vi "SLSC Add or Remove Channels.vi"(0 "Section Ref in":T1 format="%.0x", 1 "Properties":string="Properties", 2 "Command Channel":string="Commands", 3 "Physical Channels":string="Physical Channels", 5 "Property tree":string[](array[string]), 7 "Add or Remove":bool, 9 "SLSC EDS module in":T2, 11 "error in (no error)":errorcluster, 12 "Enums":T3[](array[typedef])) -> (4 "Section Ref out":T1 format="%.0x", 15 "error out":errorcluster)   [LabVIEW 2019, in "SLSC EDS System Explorer.lvlib"]
uses:
  SLSC EDS System Explorer.lvlib
  SLSC EDS API/JSON parsing/enum.ctl
  <vilib>/NI VeriStand/Custom Device API/Custom Device Item Ref.ctl
  SLSC EDS API/JSON parsing/EDSjsonStructure.ctl
  SLSC EDS API/JSON parsing/property.ctl
  SLSC EDS API/JSON parsing/command.ctl
  SLSC EDS API/JSON parsing/scale.ctl
  SLSC EDS API/JSON parsing/physicalChannel.ctl
  SLSC EDS API/JSON parsing/register.ctl
  <vilib>/NI VeriStand/Custom Device Tools/Custom Device Utility Library/NI VeriStand - Search for Item by Name.vi
  <vilib>/NI VeriStand/Custom Device Tools/Custom Device Utility Library/NI VeriStand - Search for All Items by Name.vi
  <vilib>/NI VeriStand/Custom Device Tools/Custom Device Utility Library/Custom Device Utility Library.lvlib
  <vilib>/NI VeriStand/Custom Device API/Custom Device API.lvlib
  SLSC UI API/SLSC Tree Control.lvlib
panel:
  # "not working\nregisterMap->registers->initialValue"
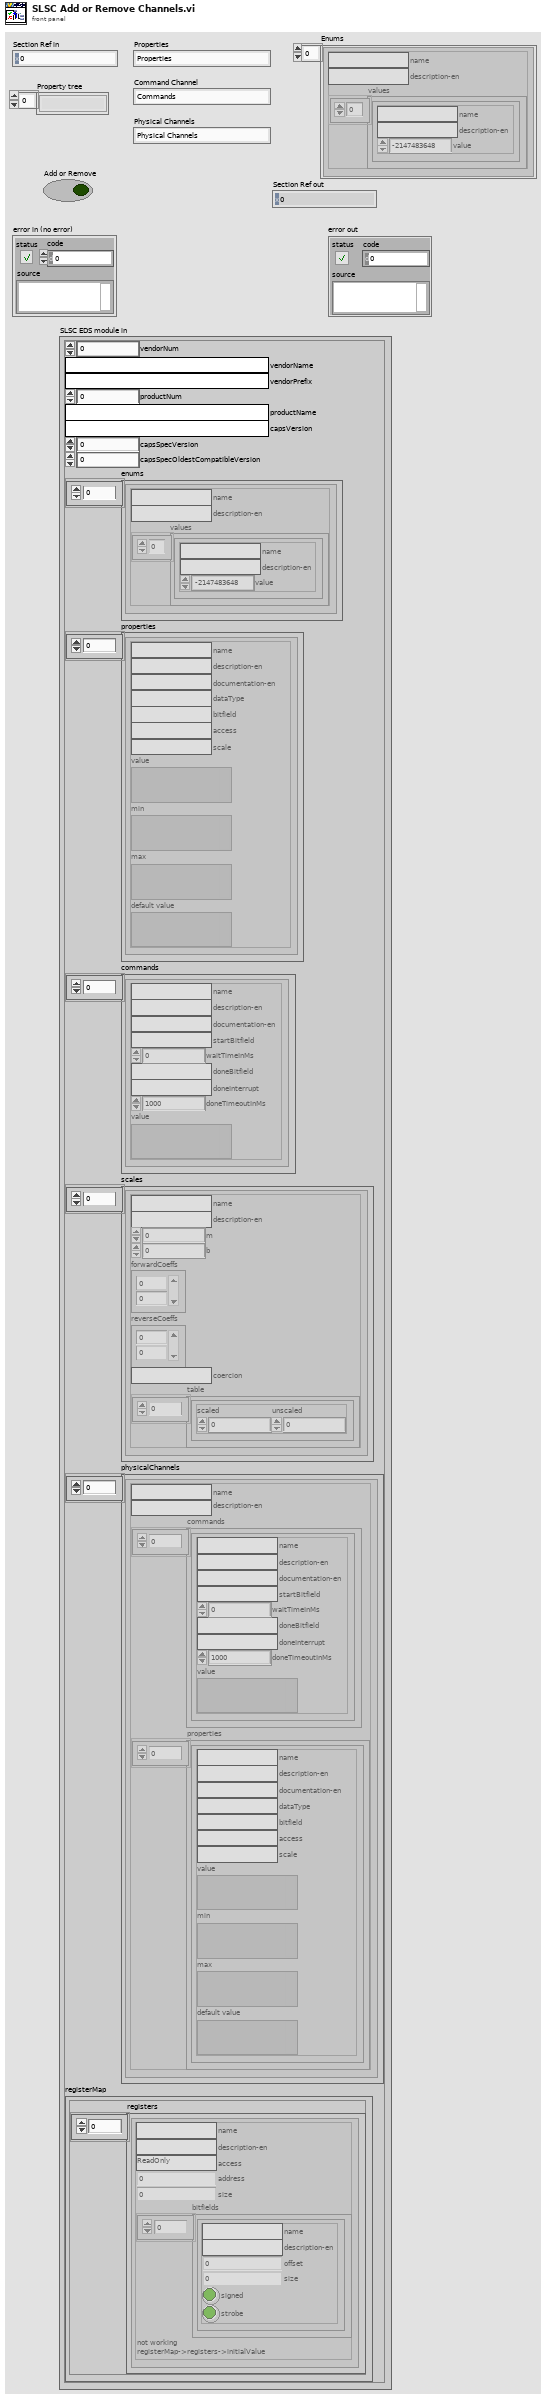
[diagram p1: front panel]
types:
  T1 = typedef "Custom Device API.lvlib/Custom Device Item Ref.ctl" = u64
  T2 = typedef "EDSjsonStructure.ctl" = cluster{"vendorNum":u32, "vendorName":string, "vendorPrefix":string, "productNum":u32, "productName":string, "capsVersion":string, "capsSpecVersion":u32, "capsSpecOldestCompatibleVersion":u32, "enums":T3[], "properties":T4[], "commands":T5[], "scales":T6[], "physicalChannels":T7[], "registerMap":cluster{"registers":T8[]}}
  T3 = typedef "enum.ctl" = cluster{"name":string, "description-en":string, "values":cluster{"name":string, "description-en":string, "value":i32}[]}
  T4 = typedef "property.ctl" = cluster{"name":string, "description-en":string, "documentation-en":string, "dataType":string, "bitfield":string, "access":string, "scale":string, "value":variant, "min":variant, "max":variant, "default value":variant}
  T5 = typedef "command.ctl" = cluster{"name":string, "description-en":string, "documentation-en":string, "startBitfield":string, "waitTimeInMs":i32, "doneBitfield":string, "doneInterrupt":string, "doneTimeoutInMs":i32, "value":variant}
  T6 = typedef "scale.ctl" = cluster{"name":string, "description-en":string, "m":dbl, "b":dbl, "forwardCoeffs":dbl[], "reverseCoeffs":dbl[], "coercion":string, "table":cluster{"scaled":dbl, "unscaled":dbl}[]}
  T7 = typedef "physicalChannel.ctl" = cluster{"name":string, "description-en":string, "commands":T5[], "properties":T4[]}
  T8 = typedef "register.ctl" = cluster{"name":string, "description-en":string, "access":string, "address":u32, "size":u32, "bitfields":cluster{"name":string, "description-en":string, "offset":u32, "size":u32, "signed":bool, "strobe":bool}[]}
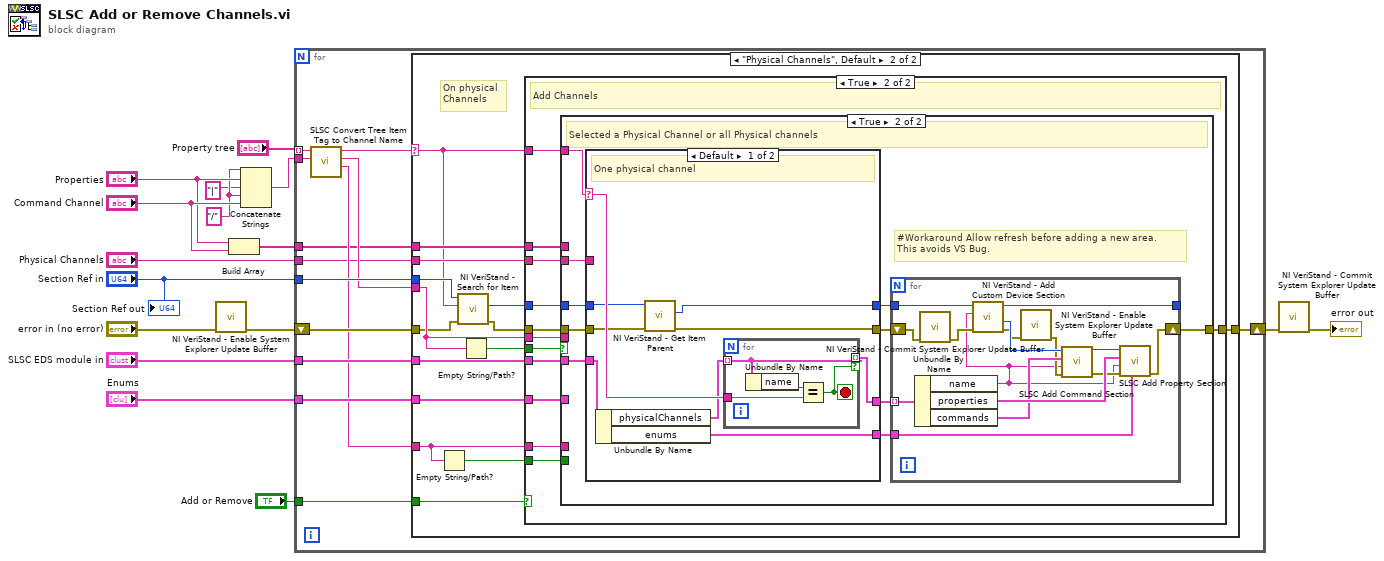
[diagram p0: block diagram]
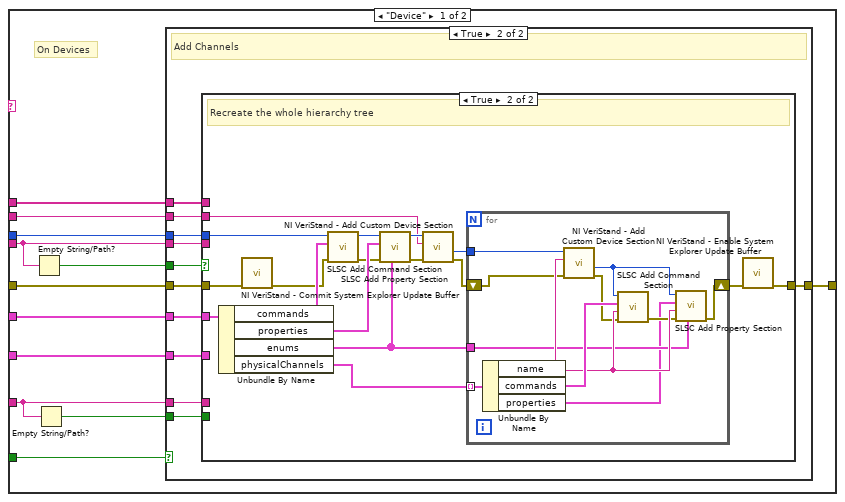
[diagram p2: hidden frame]
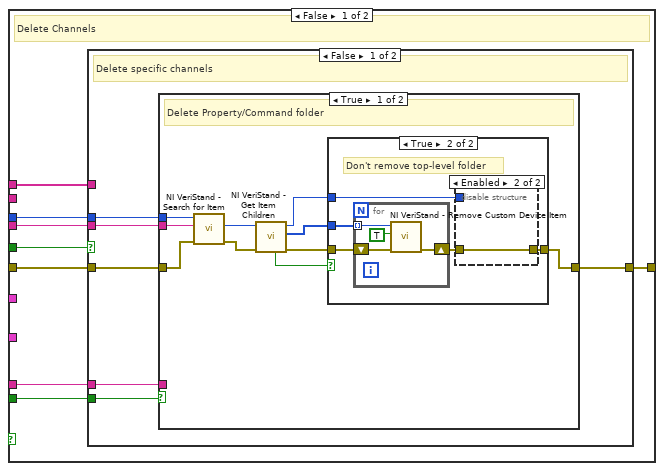
[diagram p3: hidden frame]
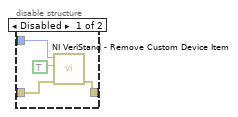
[diagram p5: hidden frame]
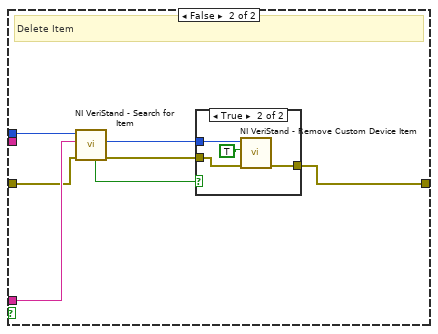
[diagram p6: hidden frame]
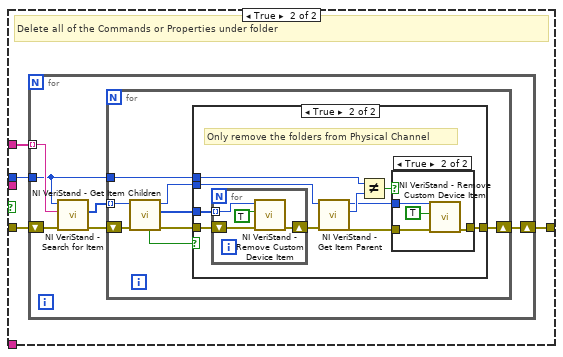
[diagram p8: hidden frame]
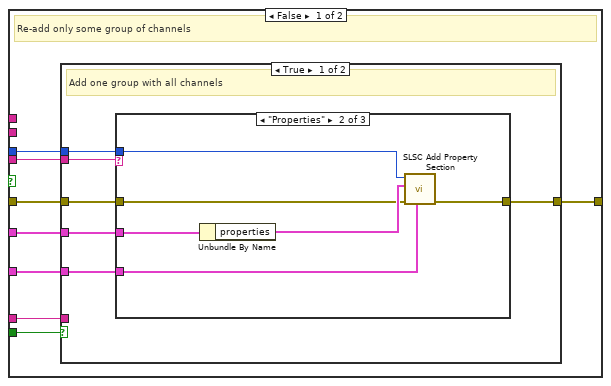
[diagram p11: hidden frame]
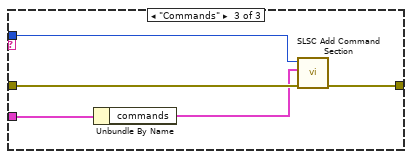
[diagram p13: hidden frame]
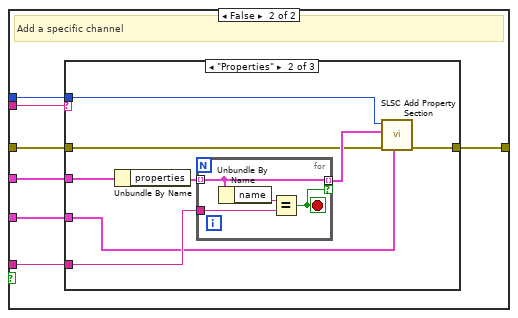
[diagram p14: hidden frame]
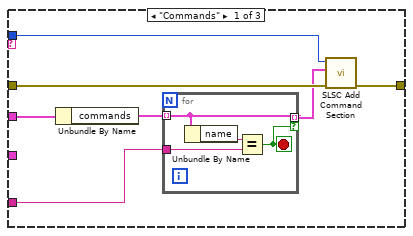
[diagram p15: hidden frame]
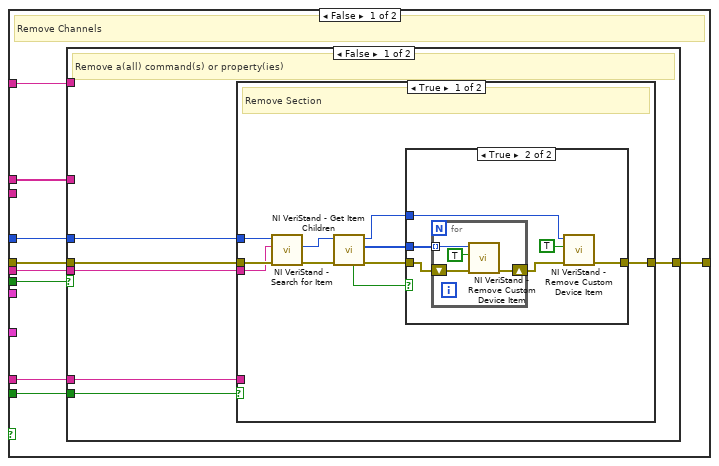
[diagram p17: hidden frame]
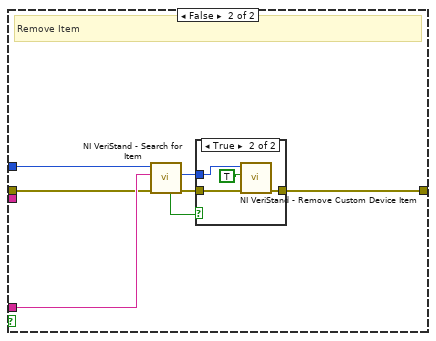
[diagram p19: hidden frame]
diagram:
  w6 = "/" ("string")
  n1 = call <vilib>:"NI VeriStand - Enable System Explorer Update Buffer.vi"("error in (no error)"="error in (no error)") -> ("error out"=w10:errorcluster)  [unwired: 10 in]
  n2 = Build Array("Properties", "Command Channel") -> (w8:string[])
  n3 = Concatenate Strings(w6, "Properties", "|" ("string"), w6, "Command Channel") -> (w4:string)
  n4 = for {
    tunnel: "Property tree" -> [w21] mode=indexing
    tunnel: w4 -> [w28]
    tunnel: "Section Ref in" -> [w27]
    shift-right: [w25] -> w15
    shift-left: w10 -> [w26]
    tunnel: "Add or Remove" -> [w24]
    tunnel: "SLSC EDS module in" -> [w23]
    tunnel: "Enums" -> [w22]
    tunnel: w8 -> [w18]
    tunnel: "Physical Channels" -> [w17]
    n5 = call "SLSC Convert Tree Item Tag to Channel Name.vi"("Type of Item"=w28, "Item String"=w21) -> ("Item Name"=w20:string, "Type of Item"=w19:string, "Device/Physical Channel"=w29:string)  [unwired: 7 in]
    n6 = case shown="\"Physical Channels\", Default" w29 {
      selector: w29 -> [_ w227]
      tunnel: w20 -> [w35 w237]
      tunnel: w27 -> [w41 w231]
      tunnel: w26 -> [w40 w229]
      tunnel: [w39 w241] -> w25
      tunnel: w24 -> [w38 w240]
      tunnel: w23 -> [w37 w239]
      tunnel: w22 -> [w36 w238]
      tunnel: w19 -> [w33 w235]
      tunnel: w18 -> [w31 w233]
      tunnel: w17 -> [w30 w232]
      frame "Device" {
        # "On Devices"
        n7 = Empty String/Path?(string/path=w33) -> (empty?=w32:bool)
        n8 = Empty String/Path?(string/path=w35) -> (empty?=w34:bool)
        n9 = case shown="True" w38 {
          tunnel: w41 -> [w49 w141]
          tunnel: w35 -> [w48 w138]
          tunnel: w40 -> [w47 w140]
          tunnel: [w46 w137] -> w39
          tunnel: w37 -> [_ w139]
          tunnel: w36 -> [_ w136]
          tunnel: w33 -> [w44 w134]
          tunnel: w34 -> [w45 w135]
          tunnel: w32 -> [w43 w133]
          tunnel: w31 -> [w42 w131]
          tunnel: w30 -> [_ w132]
          frame False {
            # "Delete Channels"
            n10 = case shown="False" w43 {
              tunnel: w49 -> [w55 w96]
              tunnel: w48 -> [w54 _]
              tunnel: w47 -> [w50 w94]
              tunnel: [w51 w93] -> w46
              tunnel: w45 -> [w53 _]
              tunnel: w44 -> [w52 _]
              tunnel: w42 -> [_ w95]
              frame False {
                # "Delete specific channels"
                n11 = case shown="True" w53 {
                  tunnel: w55 -> [w65 w87]
                  tunnel: w54 -> [_ w86]
                  tunnel: w50 -> [w64 w84]
                  tunnel: [w63 w82] -> w51
                  tunnel: w52 -> [w57 _]
                  frame True {
                    # "Delete Property/Command folder"
                    n12 = call-poly <vilib>:"NI VeriStand - Search for Item.vi"("error in"=w64, "Item Name"=w57, "Section Ref in"=w65) -> ("error out"=w59:errorcluster, "Item Ref"=w62:T1)  [unwired: 5 in, 2 out]
                    n13 = call <vilib>:"NI VeriStand - Get Item Children.vi"("error in (no error)"=w59, "Item Ref in"=w62) -> ("error out"=w58:errorcluster, "Child Refs"=w61:T1[], "Item Ref out"=w56:T1, "Found"=w60:bool)  [unwired: 6 in]
                    n14 = case shown="True" w60 {
                      tunnel: w61 -> [_ w71]
                      tunnel: w58 -> [w66 w70]
                      tunnel: [w66 w68] -> w63
                      tunnel: w56 -> [_ w67]
                      frame False {
                      }
                      frame True {
                        # "Don't remove top-level folder"
                        n15 = for {
                          tunnel: w71 -> [w80] mode=indexing
                          shift-right: [w78] -> w69
                          shift-left: w70 -> [w79]
                          n16 = call <vilib>:"NI VeriStand - Remove Custom Device Item.vi"("error in (no error)"=w79, "Force Delete (F)"=TRUE, "Item Ref in"=w80) -> ("error out"=w78:errorcluster)  [unwired: 7 in, 1 out]
                        }
                        n17 = disable-structure shown="Enabled" {
                          disable-tunnel: w69 -> [w74 w76]
                          disable-tunnel: [w73 w76] -> w68
                          disable-tunnel: w67 -> [w72 _]
                          frame Disabled {
                            n18 = call <vilib>:"NI VeriStand - Remove Custom Device Item.vi"("error in (no error)"=w74, "Force Delete (F)"=TRUE, "Item Ref in"=w72) -> ("error out"=w73:errorcluster)  [unwired: 7 in, 1 out]
                          }
                          frame Enabled {
                          }
                        }
                      }
                    }
                  }
                  frame False {
                    # "Delete Item"
                    n19 = call-poly <vilib>:"NI VeriStand - Search for Item.vi"("error in"=w84, "Item Name"=w86, "Section Ref in"=w87) -> ("error out"=w83:errorcluster, "Item Ref"=w85:T1, "Found"=w81:bool)  [unwired: 5 in, 1 out]
                    n20 = case shown="True" w81 {
                      tunnel: w85 -> [_ w92]
                      tunnel: w83 -> [w88 w91]
                      tunnel: [w88 w90] -> w82
                      frame False {
                      }
                      frame True {
                        n21 = call <vilib>:"NI VeriStand - Remove Custom Device Item.vi"("error in (no error)"=w91, "Force Delete (F)"=TRUE, "Item Ref in"=w92) -> ("error out"=w90:errorcluster)  [unwired: 7 in, 1 out]
                      }
                    }
                  }
                }
              }
              frame True {
                # "Delete all of the Commands or Properties under folder"
                n22 = for {
                  tunnel: w96 -> [w97]
                  tunnel: w95 -> [w99] mode=indexing
                  shift-right: [w98] -> w93
                  shift-left: w94 -> [w102]
                  n23 = call-poly <vilib>:"NI VeriStand - Search for Item.vi"("error in"=w102, "Item Name"=w99, "Section Ref in"=w97) -> ("error out"=w100:errorcluster, "Item Refs"=w101:T1[])  [unwired: 5 in, 2 out]
                  n24 = for {
                    tunnel: w101 -> [w110] mode=indexing
                    shift-right: [w105] -> w98
                    shift-left: w100 -> [w107]
                    tunnel: w97 -> [w103]
                    n25 = call <vilib>:"NI VeriStand - Get Item Children.vi"("error in (no error)"=w107, "Item Ref in"=w110) -> ("error out"=w106:errorcluster, "Child Refs"=w109:T1[], "Item Ref out"=w104:T1, "Found"=w108:bool)  [unwired: 6 in]
                    n26 = case shown="True" w108 {
                      tunnel: w109 -> [_ w121]
                      tunnel: w106 -> [w111 w120]
                      tunnel: [w111 w119] -> w105
                      tunnel: w104 -> [_ w118]
                      tunnel: w103 -> [_ w114]
                      frame False {
                      }
                      frame True {
                        # "Only remove the folders from Physical Channel"
                        n27 = for {
                          tunnel: w121 -> [w127] mode=indexing
                          shift-right: [w129] -> w117
                          shift-left: w120 -> [w130]
                          n28 = call <vilib>:"NI VeriStand - Remove Custom Device Item.vi"("error in (no error)"=w130, "Force Delete (F)"=TRUE, "Item Ref in"=w127) -> ("error out"=w129:errorcluster)  [unwired: 7 in, 1 out]
                        }
                        n29 = call <vilib>:"NI VeriStand - Get Item Parent.vi"("error in (no error)"=w117, "Item Ref in"=w118) -> ("error out"=w116:errorcluster, "Parent Ref"=w115:T1, "Item Ref out"=w112:T1)  [unwired: 6 in, 1 out]
                        n30 = Not Equal?(x=w114, y=w115) -> (x != y?=w113:bool)
                        n31 = case shown="True" w113 {
                          tunnel: [w122 w126] -> w119
                          tunnel: w116 -> [w122 w124]
                          tunnel: w112 -> [_ w123]
                          frame False {
                          }
                          frame True {
                            n32 = call <vilib>:"NI VeriStand - Remove Custom Device Item.vi"("error in (no error)"=w124, "Force Delete (F)"=TRUE, "Item Ref in"=w123) -> ("error out"=w126:errorcluster)  [unwired: 7 in, 1 out]
                          }
                        }
                      }
                    }
                  }
                }
              }
            }
          }
          frame True {
            # "Add Channels"
            n33 = case shown="True" w133 {
              tunnel: w141 -> [w149 w204]
              tunnel: w140 -> [w148 w202]
              tunnel: w139 -> [w147 w214]
              tunnel: w138 -> [w146 _]
              tunnel: [w145 w199] -> w137
              tunnel: w136 -> [w144 _]
              tunnel: w135 -> [w143 _]
              tunnel: w134 -> [w142 _]
              tunnel: w132 -> [_ w203]
              tunnel: w131 -> [_ _]
              frame False {
                # "Re-add only some group of channels"
                n34 = case shown="True" w143 {
                  tunnel: w149 -> [w154 w174]
                  tunnel: w148 -> [w153 w173]
                  tunnel: w147 -> [w155 w172]
                  tunnel: w146 -> [_ w171]
                  tunnel: [w152 w170] -> w145
                  tunnel: w144 -> [w151 w169]
                  tunnel: w142 -> [w150 w168]
                  frame True {
                    # "Add one group with all channels"
                    n35 = case shown="\"Properties\"" w150 {
                      tunnel: w155 -> [_ w162 w167]
                      tunnel: w154 -> [_ w160 w166]
                      tunnel: w153 -> [w156 w159 w165]
                      tunnel: [w156 w158 w164] -> w152
                      tunnel: w151 -> [_ w157 _]
                      frame Default {
                      }
                      frame "Properties" {
                        n36 = Unbundle By Name(w162) -> ("properties"=w161:T4[])
                        n37 = call "SLSC Add Property Section.vi"("enums"=w157, "error in (no error)"=w159, "properties"=w161, "Parent Ref in"=w160) -> ("error out"=w158:errorcluster)  [unwired: 6 in, 1 out]
                      }
                      frame "Commands" {
                        n38 = Unbundle By Name(w167) -> ("commands"=w163:T5[])
                        n39 = call "SLSC Add Command Section.vi"("error in (no error)"=w165, "commands"=w163, "Parent Ref in"=w166) -> ("error out"=w164:errorcluster)  [unwired: 7 in, 1 out]
                      }
                    }
                  }
                  frame False {
                    # "Add a specific channel"
                    n40 = case shown="\"Properties\"" w168 {
                      tunnel: w174 -> [w178 w190 _]
                      tunnel: w173 -> [w176 w188 w198]
                      tunnel: w172 -> [w180 w192 _]
                      tunnel: w171 -> [w179 w191 _]
                      tunnel: [w177 w187 w198] -> w170
                      tunnel: w169 -> [_ w186 _]
                      frame "Commands" {
                        n41 = Unbundle By Name(w180) -> ("commands"=w181:T5[])
                        n42 = for {
                          tunnel: w181 -> [w183] mode=indexing
                          tunnel: w179 -> [w185]
                          tunnel: [w183] -> w175 mode=indexing if=w182
                          stop <- w182 stop-if-true
                          n43 = Unbundle By Name(w183) -> ("name"=w184:string)
                          n44 = Equal?(x=w184, y=w185) -> (x = y?=w182:bool)
                        }
                        n45 = call "SLSC Add Command Section.vi"("error in (no error)"=w176, "commands"=w175, "Parent Ref in"=w178) -> ("error out"=w177:errorcluster)  [unwired: 7 in, 1 out]
                      }
                      frame "Properties" {
                        n46 = Unbundle By Name(w192) -> ("properties"=w193:T4[])
                        n47 = for {
                          tunnel: w193 -> [w195] mode=indexing
                          tunnel: w191 -> [w197]
                          tunnel: [w195] -> w189 mode=indexing if=w194
                          stop <- w194 stop-if-true
                          n48 = Unbundle By Name(w195) -> ("name"=w196:string)
                          n49 = Equal?(x=w196, y=w197) -> (x = y?=w194:bool)
                        }
                        n50 = call "SLSC Add Property Section.vi"("enums"=w186, "error in (no error)"=w188, "properties"=w189, "Parent Ref in"=w190) -> ("error out"=w187:errorcluster)  [unwired: 6 in, 1 out]
                      }
                      frame Default {
                        # "This should not happen, but if does\nit will not do any action!"
                      }
                    }
                  }
                }
              }
              frame True {
                # "Recreate the whole hierarchy tree"
                n51 = Unbundle By Name(w214) -> ("commands"=w213:T5[], "properties"=w212:T4[], "enums"=w209:T3[], "physicalChannels"=w210:T7[])
                n52 = call <vilib>:"NI VeriStand - Commit System Explorer Update Buffer.vi"("error in (no error)"=w202) -> ("error out"=w201:errorcluster)  [unwired: 10 in]
                n53 = call "SLSC Add Command Section.vi"("error in (no error)"=w201, "commands"=w213, "Parent Ref in"=w204) -> ("error out"=w211:errorcluster, "Parent Ref out"=w215:T1)  [unwired: 7 in]
                n54 = call "SLSC Add Property Section.vi"("enums"=w209, "error in (no error)"=w211, "properties"=w212, "Parent Ref in"=w215) -> ("error out"=w206:errorcluster, "Parent Ref out"=w207:T1)  [unwired: 6 in]
                n55 = call <vilib>:"NI VeriStand - Add Custom Device Section.vi"("error in (no error)"=w206, "Section Name"=w203, "Parent Ref in"=w207) -> ("error out"=w205:errorcluster, "Section Ptr"=w208:T1)  [unwired: 5 in, 2 out]
                n56 = for {
                  tunnel: w210 -> [w226] mode=indexing
                  shift-right: [w221] -> w200
                  shift-left: w205 -> [w217]
                  tunnel: w209 -> [w220]
                  tunnel: w208 -> [w224]
                  n57 = Unbundle By Name(w226) -> ("name"=w223:string, "commands"=w225:T5[], "properties"=w219:T4[])
                  n58 = call <vilib>:"NI VeriStand - Add Custom Device Section.vi"("error in (no error)"=w217, "Section Name"=w223, "Parent Ref in"=w224) -> ("error out"=w216:errorcluster, "Section Ptr"=w218:T1)  [unwired: 5 in, 2 out]
                  n59 = call "SLSC Add Command Section.vi"("error in (no error)"=w216, "Physical Channel"=w223, "commands"=w225, "Parent Ref in"=w218) -> ("error out"=w222:errorcluster)  [unwired: 6 in, 1 out]
                  n60 = call "SLSC Add Property Section.vi"("enums"=w220, "error in (no error)"=w222, "Physical Channel"=w223, "properties"=w219, "Parent Ref in"=w218) -> ("error out"=w221:errorcluster)  [unwired: 5 in, 1 out]
                }
                n61 = call <vilib>:"NI VeriStand - Enable System Explorer Update Buffer.vi"("error in (no error)"=w200) -> ("error out"=w199:errorcluster)  [unwired: 10 in]
              }
            }
          }
        }
      }
      frame "Physical Channels", Default {
        # "On physical\nChannels"
        n62 = Empty String/Path?(string/path=w237) -> (empty?=w236:bool)
        n63 = call-poly <vilib>:"NI VeriStand - Search for Item.vi"("error in"=w229, "Item Name"=w227, "Section Ref in"=w231) -> ("error out"=w228:errorcluster, "Item Ref"=w230:T1)  [unwired: 5 in, 2 out]
        n64 = Empty String/Path?(string/path=w235) -> (empty?=w234:bool)
        n65 = case shown="True" w240 {
          tunnel: w230 -> [w250 w335]
          tunnel: w237 -> [w249 w332]
          tunnel: w228 -> [w248 w334]
          tunnel: [w247 w331] -> w241
          tunnel: w239 -> [_ w333]
          tunnel: w238 -> [_ w330]
          tunnel: w235 -> [w245 w328]
          tunnel: w236 -> [w246 w329]
          tunnel: w234 -> [w244 w327]
          tunnel: w233 -> [w243 w324]
          tunnel: w227 -> [w242 w325]
          tunnel: w232 -> [_ w326]
          frame False {
            # "Remove Channels"
            n66 = case shown="False" w244 {
              tunnel: w250 -> [w251 w291]
              tunnel: w249 -> [w256 _]
              tunnel: w248 -> [w252 w290]
              tunnel: [w253 w296] -> w247
              tunnel: w246 -> [w255 _]
              tunnel: w245 -> [w254 _]
              tunnel: w243 -> [_ w295]
              tunnel: w242 -> [_ _]
              frame False {
                # "Remove a(all) command(s) or property(ies)"
                n67 = case shown="True" w255 {
                  tunnel: w251 -> [w266 w278]
                  tunnel: w256 -> [_ w284]
                  tunnel: w252 -> [w265 w282]
                  tunnel: [w264 w280] -> w253
                  tunnel: w254 -> [w258 _]
                  frame True {
                    # "Remove Section"
                    n68 = call-poly <vilib>:"NI VeriStand - Search for Item.vi"("error in"=w265, "Item Name"=w258, "Section Ref in"=w266) -> ("error out"=w260:errorcluster, "Item Ref"=w263:T1)  [unwired: 5 in, 2 out]
                    n69 = call <vilib>:"NI VeriStand - Get Item Children.vi"("error in (no error)"=w260, "Item Ref in"=w263) -> ("error out"=w259:errorcluster, "Child Refs"=w262:T1[], "Item Ref out"=w257:T1, "Found"=w261:bool)  [unwired: 6 in]
                    n70 = case shown="True" w261 {
                      tunnel: w262 -> [_ w273]
                      tunnel: w259 -> [w267 w272]
                      tunnel: [w267 w269] -> w264
                      tunnel: w257 -> [_ w271]
                      frame False {
                      }
                      frame True {
                        n71 = for {
                          tunnel: w273 -> [w277] mode=indexing
                          shift-right: [w275] -> w270
                          shift-left: w272 -> [w276]
                          n72 = call <vilib>:"NI VeriStand - Remove Custom Device Item.vi"("error in (no error)"=w276, "Force Delete (F)"=TRUE, "Item Ref in"=w277) -> ("error out"=w275:errorcluster)  [unwired: 7 in, 1 out]
                        }
                        n73 = call <vilib>:"NI VeriStand - Remove Custom Device Item.vi"("error in (no error)"=w270, "Force Delete (F)"=TRUE, "Item Ref in"=w271) -> ("error out"=w269:errorcluster)  [unwired: 7 in, 1 out]
                      }
                    }
                  }
                  frame False {
                    # "Remove Item"
                    n74 = call-poly <vilib>:"NI VeriStand - Search for Item.vi"("error in"=w282, "Item Name"=w284, "Section Ref in"=w278) -> ("error out"=w281:errorcluster, "Item Ref"=w283:T1, "Found"=w279:bool)  [unwired: 5 in, 1 out]
                    n75 = case shown="True" w279 {
                      tunnel: w283 -> [_ w289]
                      tunnel: w281 -> [w285 w288]
                      tunnel: [w285 w287] -> w280
                      frame False {
                      }
                      frame True {
                        n76 = call <vilib>:"NI VeriStand - Remove Custom Device Item.vi"("error in (no error)"=w288, "Force Delete (F)"=TRUE, "Item Ref in"=w289) -> ("error out"=w287:errorcluster)  [unwired: 7 in, 1 out]
                      }
                    }
                  }
                }
              }
              frame True {
                # "Remove all Comm/Properties"
                n77 = call <vilib>:"NI VeriStand - Get Item Children.vi"("error in (no error)"=w290, "Item Ref in"=w291) -> ("error out"=w292:errorcluster, "Child Refs"=w294:T1[], "Found"=w293:bool)  [unwired: 6 in, 1 out]
                n78 = case shown="True" w293 {
                  tunnel: w294 -> [_ w299]
                  tunnel: w292 -> [w297 w300]
                  tunnel: [w297 w301] -> w296
                  tunnel: w295 -> [_ w298]
                  frame False {
                  }
                  frame True {
                    n79 = for {
                      shift-right: [w305] -> w301
                      shift-left: w300 -> [w304]
                      tunnel: w299 -> [w303] mode=indexing
                      tunnel: w298 -> [w302]
                      n80 = for {
                        tunnel: w303 -> [w307]
                        tunnel: w302 -> [w306] mode=indexing
                        shift-right: [w311] -> w305
                        shift-left: w304 -> [w309]
                        n81 = call-poly <vilib>:"NI VeriStand - Search for Item.vi"("error in"=w309, "Item Name"=w306, "Section Ref in"=w307) -> ("error out"=w308:errorcluster, "Item Refs"=w310:T1[])  [unwired: 5 in, 2 out]
                        n82 = for {
                          tunnel: w310 -> [w318] mode=indexing
                          shift-right: [w314] -> w311
                          shift-left: w308 -> [w319]
                          n83 = call <vilib>:"NI VeriStand - Get Item Children.vi"("error in (no error)"=w319, "Item Ref in"=w318) -> ("error out"=w317:errorcluster, "Child Refs"=w316:T1[], "Item Ref out"=w312:T1)  [unwired: 6 in, 1 out]
                          n84 = for {
                            shift-right: [w323] -> w313
                            shift-left: w317 -> [w321]
                            tunnel: w316 -> [w320] mode=indexing
                            n85 = call <vilib>:"NI VeriStand - Remove Custom Device Item.vi"("error in (no error)"=w321, "Force Delete (F)"=TRUE, "Item Ref in"=w320) -> ("error out"=w323:errorcluster)  [unwired: 7 in, 1 out]
                          }
                          n86 = call <vilib>:"NI VeriStand - Remove Custom Device Item.vi"("error in (no error)"=w313, "Force Delete (F)"=TRUE, "Item Ref in"=w312) -> ("error out"=w314:errorcluster)  [unwired: 7 in, 1 out]
                        }
                      }
                    }
                  }
                }
              }
            }
          }
          frame True {
            # "Add Channels"
            n87 = case shown="True" w327 {
              tunnel: w335 -> [w340 w426]
              tunnel: w334 -> [w341 w428]
              tunnel: w333 -> [w343 w433]
              tunnel: w332 -> [w338 _]
              tunnel: [w344 w432] -> w331
              tunnel: w330 -> [w342 _]
              tunnel: w329 -> [w336 _]
              tunnel: w328 -> [w339 _]
              tunnel: w326 -> [_ w424]
              tunnel: w325 -> [w337 w425]
              tunnel: w324 -> [_ _]
              frame False {
                # "Selected a item under a Physical Channel"
                n88 = case shown="False" w336 {
                  tunnel: w340 -> [w350 w385]
                  tunnel: w341 -> [w349 w384]
                  tunnel: w343 -> [w351 w383]
                  tunnel: w338 -> [_ w382]
                  tunnel: [w348 w381] -> w344
                  tunnel: w342 -> [w347 w380]
                  tunnel: w339 -> [w346 w379]
                  tunnel: w337 -> [w345 w378]
                  frame True {
                    # "Group of properties or commands"
                    n89 = case shown="\"Properties\"" w346 {
                      tunnel: w351 -> [_ w360 w373]
                      tunnel: w350 -> [_ w359 w372]
                      tunnel: w349 -> [w352 w358 w371]
                      tunnel: [w352 w357 w370] -> w348
                      tunnel: w347 -> [_ _ _]
                      tunnel: w345 -> [_ w355 w368]
                      frame Default {
                        # "By-pass Just in case something is not right with the tree..."
                      }
                      frame "Commands" {
                        n90 = Unbundle By Name(w360) -> ("physicalChannels"=w356:T7[])
                        n91 = for {
                          tunnel: w356 -> [w362] mode=indexing
                          tunnel: w355 -> [w364]
                          tunnel: [w362] -> w354 if=w361
                          stop <- w361 stop-if-true
                          n92 = Unbundle By Name(w362) -> ("name"=w363:string)
                          n93 = Equal?(x=w363, y=w364) -> (x = y?=w361:bool)
                        }
                        n94 = Unbundle By Name(w354) -> ("commands"=w353:T5[])
                        n95 = call "SLSC Add Command Section.vi"("error in (no error)"=w358, "Physical Channel"=w355, "commands"=w353, "Parent Ref in"=w359) -> ("error out"=w357:errorcluster)  [unwired: 6 in, 1 out]
                      }
                      frame "Properties" {
                        n96 = Unbundle By Name(w373) -> ("physicalChannels"=w369:T7[], "enums"=w365:T3[])
                        n97 = for {
                          tunnel: w369 -> [w375] mode=indexing
                          tunnel: w368 -> [w377]
                          tunnel: [w375] -> w367 if=w374
                          stop <- w374 stop-if-true
                          n98 = Unbundle By Name(w375) -> ("name"=w376:string)
                          n99 = Equal?(x=w376, y=w377) -> (x = y?=w374:bool)
                        }
                        n100 = Unbundle By Name(w367) -> ("properties"=w366:T4[])
                        n101 = call "SLSC Add Property Section.vi"("enums"=w365, "error in (no error)"=w371, "Physical Channel"=w368, "properties"=w366, "Parent Ref in"=w372) -> ("error out"=w370:errorcluster)  [unwired: 5 in, 1 out]
                      }
                    }
                  }
                  frame False {
                    # "Specific element on the channel"
                    n102 = case shown="\"Properties\"" w379 {
                      tunnel: w385 -> [w394 w412 _]
                      tunnel: w384 -> [w393 w411 w423]
                      tunnel: w383 -> [w395 w413 _]
                      tunnel: w382 -> [w386 w406 _]
                      tunnel: [w392 w410 w423] -> w381
                      tunnel: w380 -> [w391 _ _]
                      tunnel: w378 -> [w387 w405 _]
                      frame "Properties" {
                        # "Add specific property under the channel"
                        n103 = Unbundle By Name(w395) -> ("physicalChannels"=w396:T7[])
                        n104 = for {
                          tunnel: w396 -> [w402] mode=indexing
                          tunnel: w387 -> [w404]
                          tunnel: [w402] -> w389 if=w401
                          stop <- w401 stop-if-true
                          n105 = Unbundle By Name(w402) -> ("name"=w403:string)
                          n106 = Equal?(x=w403, y=w404) -> (x = y?=w401:bool)
                        }
                        n107 = Unbundle By Name(w389) -> ("properties"=w390:T4[])
                        n108 = for {
                          tunnel: w390 -> [w398] mode=indexing
                          tunnel: w386 -> [w400]
                          tunnel: [w398] -> w388 mode=indexing if=w397
                          stop <- w397 stop-if-true
                          n109 = Unbundle By Name(w398) -> ("name"=w399:string)
                          n110 = Equal?(x=w399, y=w400) -> (x = y?=w397:bool)
                        }
                        n111 = call "SLSC Add Property Section.vi"("enums"=w391, "error in (no error)"=w393, "Physical Channel"=w387, "properties"=w388, "Parent Ref in"=w394) -> ("error out"=w392:errorcluster)  [unwired: 5 in, 1 out]
                      }
                      frame "Commands" {
                        # "Add specific command under the channel"
                        n112 = Unbundle By Name(w413) -> ("physicalChannels"=w414:T7[])
                        n113 = for {
                          tunnel: w414 -> [w420] mode=indexing
                          tunnel: w405 -> [w422]
                          tunnel: [w420] -> w408 if=w419
                          stop <- w419 stop-if-true
                          n114 = Unbundle By Name(w420) -> ("name"=w421:string)
                          n115 = Equal?(x=w421, y=w422) -> (x = y?=w419:bool)
                        }
                        n116 = Unbundle By Name(w408) -> ("commands"=w409:T5[])
                        n117 = for {
                          tunnel: w409 -> [w416] mode=indexing
                          tunnel: w406 -> [w418]
                          tunnel: [w416] -> w407 mode=indexing if=w415
                          stop <- w415 stop-if-true
                          n118 = Unbundle By Name(w416) -> ("name"=w417:string)
                          n119 = Equal?(x=w417, y=w418) -> (x = y?=w415:bool)
                        }
                        n120 = call "SLSC Add Command Section.vi"("error in (no error)"=w411, "Physical Channel"=w405, "commands"=w407, "Parent Ref in"=w412) -> ("error out"=w410:errorcluster)  [unwired: 6 in, 1 out]
                      }
                      frame Default {
                        # "Ops... something was wrong..."
                      }
                    }
                  }
                }
              }
              frame True {
                # "#Workaround Allow refresh before adding a new area.\nThis avoids VS Bug."
                # "Selected a Physical Channel or all Physical channels"
                n121 = case shown="Default" w425 {
                  selector: w425 -> [w441 _]
                  tunnel: w433 -> [w442 w451]
                  tunnel: [w439 w450] -> w431
                  tunnel: [w438 w449] -> w430
                  tunnel: [w436 w447] -> w429
                  tunnel: w428 -> [w437 w447]
                  tunnel: [w434 w448] -> w427
                  tunnel: w426 -> [w435 w448]
                  tunnel: w424 -> [_ _]
                  frame Default {
                    # "One physical channel"
                    n122 = Unbundle By Name(w442) -> ("physicalChannels"=w440:T7[], "enums"=w438:T3[])
                    n123 = call <vilib>:"NI VeriStand - Get Item Parent.vi"("error in (no error)"=w437, "Item Ref in"=w435) -> ("error out"=w436:errorcluster, "Parent Ref"=w434:T1)  [unwired: 6 in, 2 out]
                    n124 = for {
                      tunnel: w440 -> [w444] mode=indexing
                      tunnel: w441 -> [w446]
                      tunnel: [w444] -> w439 mode=indexing if=w443
                      stop <- w443 stop-if-true
                      n125 = Unbundle By Name(w444) -> ("name"=w445:string)
                      n126 = Equal?(x=w445, y=w446) -> (x = y?=w443:bool)
                    }
                  }
                  frame "Physical Channels" {
                    # "All Physical Channels"
                    n127 = Unbundle By Name(w451) -> ("physicalChannels"=w450:T7[], "enums"=w449:T3[])
                  }
                }
                n128 = for {
                  tunnel: w431 -> [w466] mode=indexing
                  shift-right: [w460] -> w432
                  shift-left: w429 -> [w456]
                  tunnel: w427 -> [w463]
                  tunnel: [w462] -> _
                  tunnel: w430 -> [w457]
                  n129 = Unbundle By Name(w466) -> ("name"=w452:string, "properties"=w465:T4[], "commands"=w464:T5[])
                  n130 = call <vilib>:"NI VeriStand - Commit System Explorer Update Buffer.vi"("error in (no error)"=w456) -> ("error out"=w455:errorcluster)  [unwired: 10 in]
                  n131 = call <vilib>:"NI VeriStand - Add Custom Device Section.vi"("error in (no error)"=w455, "Section Name"=w452, "Parent Ref in"=w463) -> ("error out"=w454:errorcluster, "Section Ptr"=w459:T1, "Parent Ref out"=w462:T1)  [unwired: 5 in, 1 out]
                  n132 = call <vilib>:"NI VeriStand - Enable System Explorer Update Buffer.vi"("error in (no error)"=w454) -> ("error out"=w453:errorcluster)  [unwired: 10 in]
                  n133 = call "SLSC Add Command Section.vi"("error in (no error)"=w453, "Physical Channel"=w452, "commands"=w464, "Parent Ref in"=w459) -> ("error out"=w461:errorcluster, "Parent Ref out"=w458:T1)  [unwired: 6 in]
                  n134 = call "SLSC Add Property Section.vi"("enums"=w457, "error in (no error)"=w461, "Physical Channel"=w452, "properties"=w465, "Parent Ref in"=w458) -> ("error out"=w460:errorcluster)  [unwired: 5 in, 1 out]
                }
              }
            }
          }
        }
      }
    }
  }
  n135 = call <vilib>:"NI VeriStand - Commit System Explorer Update Buffer.vi"("error in (no error)"=w15) -> ("error out"=→"error out":errorcluster)  [unwired: 10 in]
  "Section Ref out" <- "Section Ref in"
